vi "PanelManager_Create.vi"(8 "error in (no error)":errorcluster, 9 "Panel Name":string, 10 "VI Refnum":refnum<vi>, 11 "PanelManager in":refnum<class "PanelManager.lvclass">) -> (0 "error out":errorcluster, 3 "PanelManager out":refnum<class "PanelManager.lvclass">)   [LabVIEW 2015, in "PanelManager.lvclass"]
uses:
  PanelManager.lvclass
  PanelManager.lvclass/PanelManager.ctl
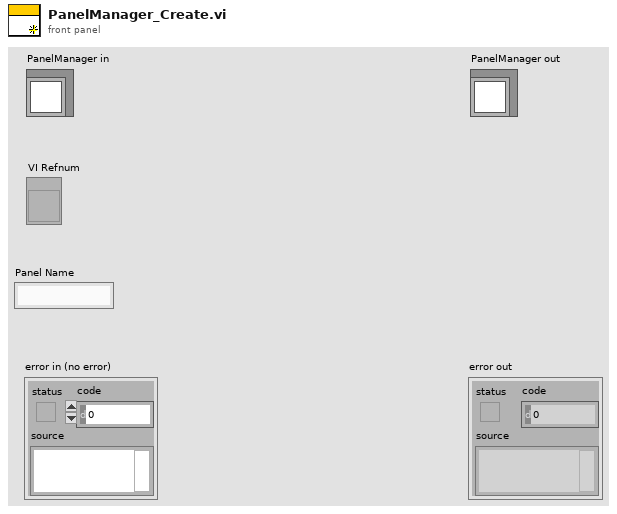
[diagram p1: front panel]
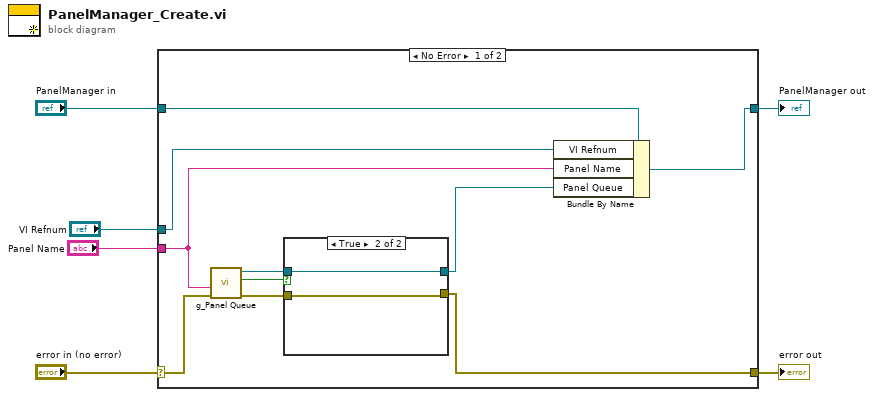
[diagram p0: block diagram]
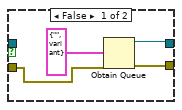
[diagram p2: hidden frame]
diagram:
  n1 = case shown="No Error" "error in (no error)" {
    selector: "error in (no error)" -> [w13 w24]
    tunnel: [w7 w24] -> w5
    tunnel: [w8 w23] -> w3
    tunnel: "PanelManager in" -> [w16 w23]
    tunnel: "VI Refnum" -> [w15 _]
    tunnel: "Panel Name" -> [w14 _]
    frame No Error {
      n2 = call "g_Panel Queue.vi"("error in (no error)"=w13, "PanelName(\"\")"=w14) -> ("error out"=w11:errorcluster, "Find?(False)"=w12:bool, "Queue Out"=w10:refnum<queue>)  [unwired: 7 in]
      n3 = case shown="True" w12 {
        tunnel: w11 -> [w19 w21]
        tunnel: w10 -> [_ w22]
        tunnel: [w18 w22] -> w9
        tunnel: [w17 w21] -> w7
        frame False {
          n4 = Obtain Queue(element data type=cluster{"cmd":string, "data":variant} {"cmd"="", "data"=variant} ("element"), error in (no error)=w19) -> (queue out=w18:refnum<queue>, error out=w17:errorcluster)  [unwired: 3 in, 1 out]
        }
        frame True {
        }
      }
      n5 = Bundle By Name(cluster=w16, "VI Refnum"=w15, "Panel Name"=w14, "Panel Queue"=w9) -> (w8:refnum<class "PanelManager.lvclass">)
    }
    frame Error {
    }
  }
  "error out" <- w5
  "PanelManager out" <- w3
